vi "Tosca-Monitor Trial-State-Rep.vi"(0 "DI":bool[](array[boolean]), 7 "Trial/State/Rep In":bool[](array[boolean]), 11 "State In":i32) -> (4 "State change?":bool, 8 "Trial/State/Rep Out":bool[](array[boolean]), 10 "Any change":bool, 15 "State Out":i32)   [LabVIEW 2020]
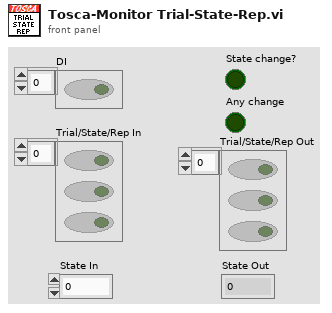
[diagram p1: front panel]
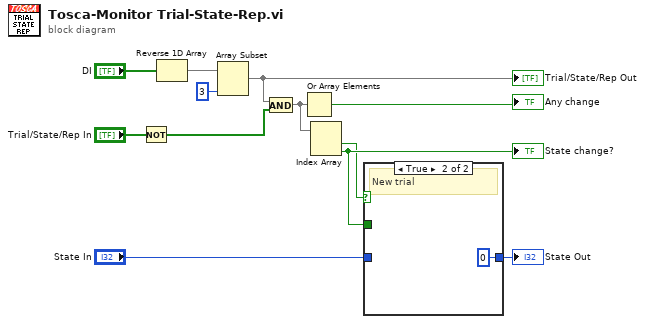
[diagram p0: block diagram]
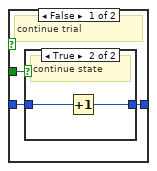
[diagram p2: hidden frame]
diagram:
  n1 = Not(x="Trial/State/Rep In") -> (.not. x?=w7:bool[])
  n2 = Reverse 1D Array(array="DI") -> (reversed array=w11:bool[])
  n3 = Array Subset(array=w11, length=3) -> (w9:bool[])  [unwired: 1 in]
  "Trial/State/Rep Out" <- w9
  n4 = And(x=w9, y=w7) -> (x .and. y?=w5:bool[])
  n5 = Or Array Elements(Boolean array=w5) -> (logical OR=→"Any change":bool)
  n6 = Index Array(array=w5) -> (element #1=w1:bool, element #2=w2:bool)  [unwired: 2 in]
  "State change?" <- w2
  n7 = case shown="True" w1 {
    tunnel: "State In" -> [w15 _]
    tunnel: [w14 0 ("State In")] -> w3
    tunnel: w2 -> [w13 _]
    frame False {
      # "continue trial"
      n8 = case shown="True" w13 {
        tunnel: w15 -> [w16 w18]
        tunnel: [w16 w17] -> w14
        frame False {
          # "new state"
        }
        frame True {
          # "continue state"
          n9 = Increment(x=w18) -> (x+1=w17:i32)
        }
      }
    }
    frame True {
      # "New trial"
    }
  }
  "State Out" <- w3
